vi "StatePowerManagement.vi"(0 "Master State":enum16{"Normal", "Climb"}(ring)) -> ()   [LabVIEW 2020]
doc: "This VI decides whether or not power should be diverted away from non-critical subsystems in an emergency or during certain periods of the match."
uses:
  GlobalMiscellaneous.vi
  sensordata.vi
  GlobalDriverStationData.vi
  <vilib>/Rock Robotics/WPI/DriverStation/WPI_DriverStationRobotMode2.ctl
  GlobalDrivebase.vi
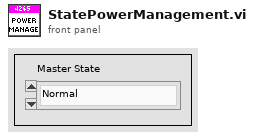
[diagram p1: front panel]
types:
  T1 = typedef "WPI_DriverStationRobotMode2.ctl" = enum16{"Autonomous Disabled", "Autonomous Enabled", "Teleop Disabled", "Teleop Enabled", "Disconnected", "Finish", "Test Disabled", "Test Enabled", "Emergency Stopped"}
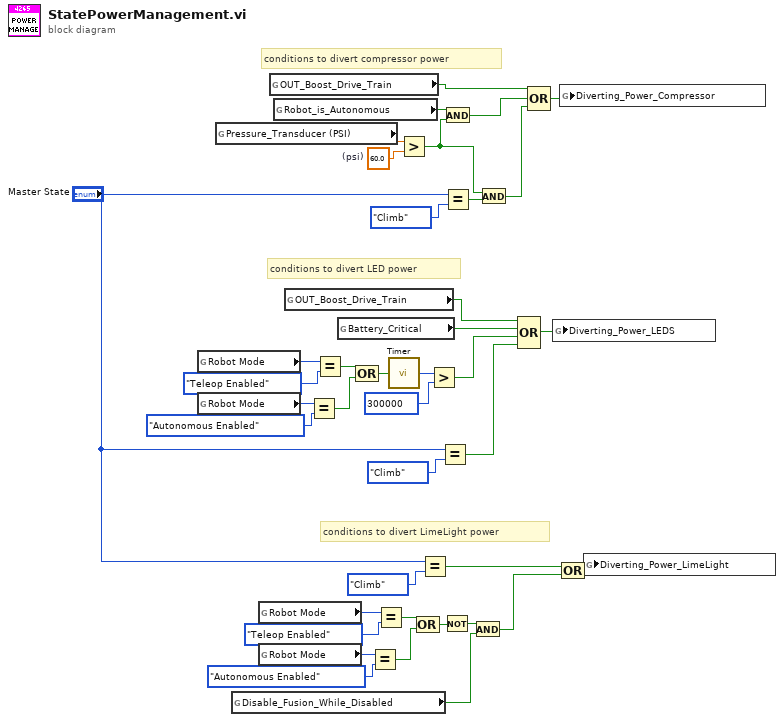
[diagram p0: block diagram]
diagram:
  w25 = 60.0  # (psi)
  # "conditions to divert LimeLight power"
  # "conditions to divert LED power"
  # "conditions to divert compressor power"
  n1 = global read "GlobalDriverStationData.vi" "Robot Mode"() -> (w36:T1)
  n2 = global read "GlobalDriverStationData.vi" "Robot Mode"() -> (w33:T1)
  n3 = global read "sensordata.vi" "Pressure_Transducer (PSI)"() -> (w24:dbl)
  n4 = global read "GlobalDriverStationData.vi" "Disable_Fusion_While_Disabled"() -> (w4:bool)
  n5 = global read "GlobalDriverStationData.vi" "Robot Mode"() -> (w12:T1)
  n6 = global read "GlobalDriverStationData.vi" "Robot Mode"() -> (w9:T1)
  n7 = global read "GlobalDrivebase.vi" "OUT_Boost_Drive_Train"() -> (w1:bool)
  n8 = global read "GlobalDriverStationData.vi" "Robot_is_Autonomous"() -> (w27:bool)
  n9 = global read "GlobalDrivebase.vi" "OUT_Boost_Drive_Train"() -> (w2:bool)
  n10 = Equal?(x=w33, y=WPI_DriverStationRobotMode2."Autonomous Enabled") -> (x = y?=w31:bool)
  n11 = Equal?(x=w36, y=WPI_DriverStationRobotMode2."Teleop Enabled") -> (x = y?=w34:bool)
  n12 = global read "sensordata.vi" "Battery_Critical"() -> (w37:bool)
  n13 = Compound Arithmetic op=OR(w34, w31) -> (w28:bool)
  n14 = Equal?(x=w9, y=WPI_DriverStationRobotMode2."Autonomous Enabled") -> (x = y?=w7:bool)
  n15 = Equal?(x=w12, y=WPI_DriverStationRobotMode2."Teleop Enabled") -> (x = y?=w10:bool)
  n16 = call "Timer.vi"("Reset Timer"=w28) -> ("Time (ms)"=w30:u32)
  n17 = Greater?(x=w24, y=w25) -> (0:w19:bool)
  n18 = Compound Arithmetic op=OR(w10, w7) -> (w6:bool)
  n19 = Equal?(x="Master State", y=enum16{"Normal", "Climb"}."Climb") -> (x = y?=w15:bool)
  n20 = Greater?(x=w30, y=u32 300000 ("x")) -> (0:w13:bool)
  n21 = Equal?(x="Master State", y=enum16{"Normal", "Climb"}."Climb") -> (x = y?=w22:bool)
  n22 = Not(x=w6) -> (.not. x?=w5:bool)
  n23 = And(x=w27, y=w19) -> (x .and. y?=w26:bool)
  n24 = Equal?(x="Master State", y=enum16{"Normal", "Climb"}."Climb") -> (x = y?=w20:bool)
  n25 = And(x=w5, y=w4) -> (x .and. y?=w3:bool)
  n26 = And(x=w19, y=w20) -> (x .and. y?=w18:bool)
  n27 = Compound Arithmetic op=OR(w2, w37, w13, w22) -> (w38:bool)
  n28 = Compound Arithmetic op=OR(w1, w26, w18) -> (w39:bool)
  n29 = global write "GlobalMiscellaneous.vi" "Diverting_Power_LEDS"(w38) -> ()
  n30 = global write "GlobalMiscellaneous.vi" "Diverting_Power_Compressor"(w39) -> ()
  n31 = Compound Arithmetic op=OR(w15, w3) -> (w17:bool)
  n32 = global write "GlobalMiscellaneous.vi" "Diverting_Power_LimeLight"(w17) -> ()
